vi "Stitch.vi"(10 "Array":picture[][](array[picture]), 11 "Map.lvclass":refnum<class "Map.lvclass">) -> (2 "Value":picture, 3 "output cluster":refnum<class "Map.lvclass">)   [LabVIEW 2016, in "Map.lvclass"]
uses:
  Map.lvclass
  <vilib>/Utility/miscctls.llb/LVBoundsTypeDef.ctl
  Map.lvclass/Map.ctl
panel:
  in  "subset rect":T1
  out "New Picture Height":i32
  out "New Picture Width":i32
  in  "new picture":picture
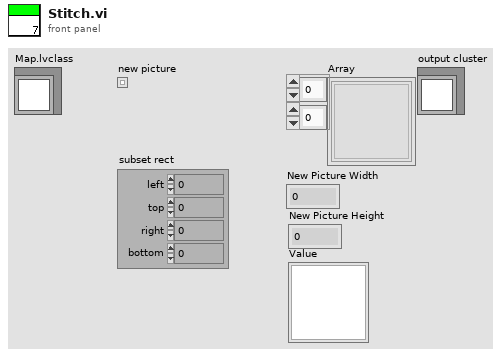
[diagram p1: front panel]
types:
  T1 = cluster{"left":i16, "top":i16, "right":i16, "bottom":i16}
  T2 = typedef "LVBoundsTypeDef.ctl" = cluster{"Width":u32, "Height":u32}
  T3 = typedef "imagedata.ctl" = cluster{"image type":i32, "image depth":i32, "image":u8[], "mask":u8[], "colors":u32[], "Rectangle":cluster{"left":i16, "top":i16, "right":i16, "bottom":i16}}
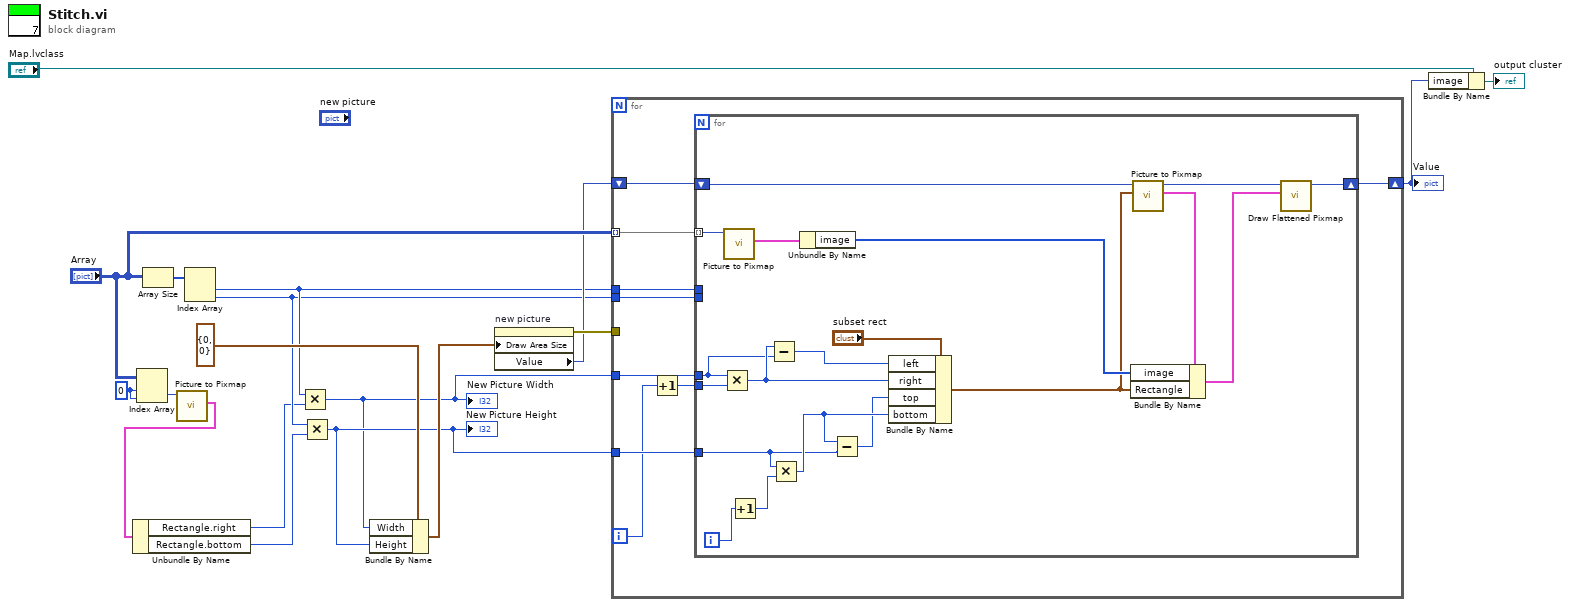
[diagram p0: block diagram]
diagram:
  w16 = 0 ("index (row)")
  n1 = Index Array(array="Array", index (row)=w16, index (col)=w16) -> (element=w15:picture)
  n2 = Array Size(array="Array") -> (size(s)=w18:i32[])
  n3 = call <vilib>:"Picture to Pixmap.vi"("picture"=w15) -> ("image data"=w14:T3)  [unwired: 9 in, 1 out]
  n4 = Unbundle By Name(w14) -> ("Rectangle.right"=w7:i16, "Rectangle.bottom"=w8:i16)
  n5 = Index Array(array=w18) -> (element #1=w10:i32, element #2=w9:i32)  [unwired: 2 in]
  n6 = Multiply(x=w10, y=w7) -> (x*y=w4:i32)
  "New Picture Width" <- w4
  n7 = Multiply(x=w9, y=w8) -> (x*y=w5:i32)
  "New Picture Height" <- w5
  n8 = Bundle By Name(cluster=T2 {"Width"=0, "Height"=0} ("Draw Area Size"), "Width"=w4, "Height"=w5) -> (w6:T2)
  n9 = property on="new picture" class="Pict"("Draw Area Size"=w6) -> (error out=w13:errorcluster, "Value"=w12:picture)  [unwired: 2 in, 1 out]
  n10 = for {
    tunnel: "Array" -> [w27] mode=indexing
    shift-right: [w25] -> w2
    shift-left: w12 -> [w26]
    tunnel: w10 -> [w24]
    tunnel: w9 -> [w23]
    tunnel: w13 -> [_]
    tunnel: w5 -> [w22]
    tunnel: w4 -> [w21]
    i -> [w20]
    n11 = Increment(x=w20) -> (x+1=w19:i32)
    n12 = for {
      tunnel: w27 -> [w46] mode=indexing
      shift-right: [w45] -> w25
      shift-left: w26 -> [w44]
      tunnel: w24 -> [_]
      tunnel: w23 -> [_]
      tunnel: w22 -> [w29]
      tunnel: w21 -> [w34]
      tunnel: w19 -> [w36]
      i -> [w32]
      n13 = Multiply(x=w34, y=w36) -> (x*y=w35:i32)
      n14 = call <vilib>:"Picture to Pixmap.vi"("picture"=w46) -> ("image data"=w39:T3)  [unwired: 9 in, 1 out]
      n15 = Increment(x=w32) -> (x+1=w31:i32)
      n16 = Subtract(x=w35, y=w34) -> (x-y=w33:i32)
      n17 = Multiply(x=w29, y=w31) -> (x*y=w30:i32)
      n18 = Unbundle By Name(w39) -> ("image"=w38:u8[])
      n19 = Subtract(x=w30, y=w29) -> (x-y=w28:i32)
      n20 = Bundle By Name(cluster="subset rect", "left"=w33, "right"=w35, "top"=w28, "bottom"=w30) -> (w37:T1)
      n21 = call <vilib>:"Picture to Pixmap.vi"("rect"=w37, "picture"=w44) -> ("image data"=w43:T3, "new picture"=w41:picture)  [unwired: 8 in]
      n22 = Bundle By Name(cluster=w43, "image"=w38, "Rectangle"=w37) -> (w40:T3)
      n23 = call <vilib>:"Draw Flattened Pixmap.vi"("image data"=w40, "picture"=w41) -> ("new picture"=w45:picture)  [unwired: 7 in]
    }
  }
  "Value" <- w2
  n24 = Bundle By Name(cluster="Map.lvclass", "image"=w2) -> (→"output cluster":refnum<class "Map.lvclass">)
